vi "CheckUserFiles.vi"(8 "ErrorArray":errorcluster[](array[cluster]), 11 "Config in":refnum<class "Config.lvclass">) -> (0 "ErrorArray":errorcluster[](array[cluster]), 3 "Config out":refnum<class "Config.lvclass">)   [LabVIEW 2014, in "Framework.lvlib" / "Config.lvclass"]
uses:
  Config.lvclass
  Config.lvclass/Config.ctl
  Accessors/Read PARTF Root Directory.vi
  <userlib>/NIST/NISTErrorLib/NISTErrorLib.lvlib
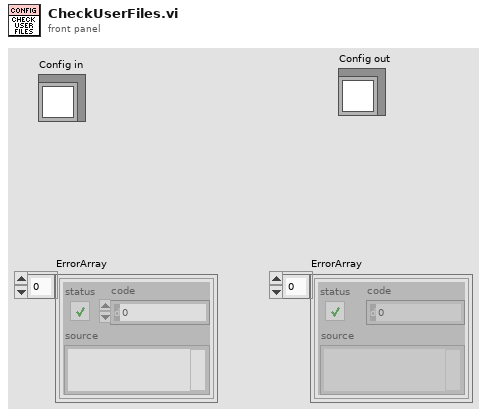
[diagram p1: front panel]
types:
  T1 = typedef "Framework.lvlib/Config.lvclass/RootDir.ctl" = cluster{"pathRootDir":path, "btnOutPath":bool, "OutDir":string, "btnOpenOutputDir":bool, "ScriptDir":string, "btnOpenScriptDir":bool, "TestDir":string, "btnOpenTestDir":bool}
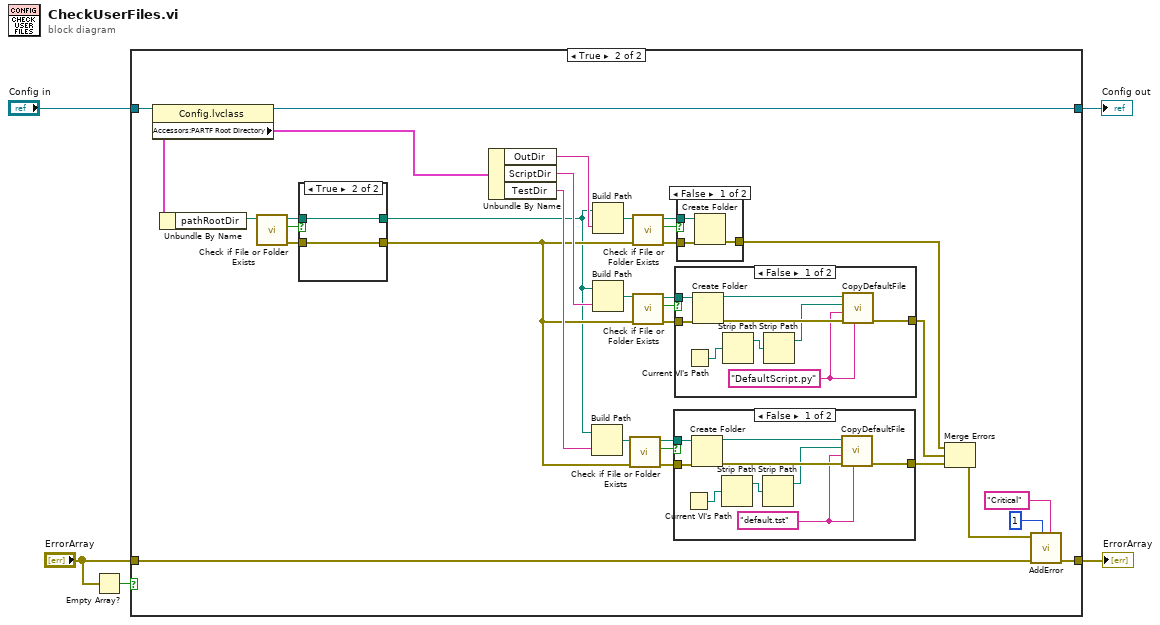
[diagram p0: block diagram]
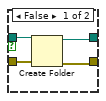
[diagram p3: hidden frame]
diagram:
  n1 = Empty Array?(array="ErrorArray") -> (empty?=w2:bool)
  n2 = case shown="True" w2 {
    tunnel: [w7 w38] -> w4
    tunnel: "Config in" -> [w7 w39]
    tunnel: "ErrorArray" -> [w6 w8]
    tunnel: [w6 w12] -> w1
    frame False {
    }
    frame True {
      n3 = property class="Config.lvclass"(reference=w39) -> (reference out=w38:refnum<class "Config.lvclass">, "Accessors:PARTF Root Directory"=w37:T1)  [unwired: 1 in, 1 out]
      n4 = Unbundle By Name(w37) -> ("pathRootDir"=w36:path)
      n5 = call <vilib>:"Check if File or Folder Exists.vi"("path"=w36) -> ("error out"=w16:errorcluster, "file or folder exists?"=w18:bool, "dup path"=w17:path)  [unwired: 8 in]
      n6 = case shown="True" w18 {
        tunnel: w17 -> [w42 w44]
        tunnel: w16 -> [w43 w45]
        tunnel: [w40 w45] -> w15
        tunnel: [w41 w44] -> w14
        frame False {
          n7 = Create Folder(path (use dialog)=w42, error in=w43) -> (created path=w41:path, error out=w40:errorcluster)  [unwired: 1 in, 1 out]
        }
        frame True {
        }
      }
      n8 = Unbundle By Name(w37) -> ("OutDir"=w35:string, "ScriptDir"=w34:string, "TestDir"=w33:string)
      n9 = Build Path(base path=w14, name or relative path=w33) -> (appended path=w30:path)
      n10 = Build Path(base path=w14, name or relative path=w35) -> (appended path=w32:path)
      n11 = Build Path(base path=w14, name or relative path=w34) -> (appended path=w31:path)
      n12 = call <vilib>:"Check if File or Folder Exists.vi"("error in (no error)"=w15, "path"=w30) -> ("error out"=w22:errorcluster, "file or folder exists?"=w13:bool, "dup path"=w23:path)  [unwired: 7 in]
      n13 = call <vilib>:"Check if File or Folder Exists.vi"("error in (no error)"=w15, "path"=w32) -> ("error out"=w27:errorcluster, "file or folder exists?"=w29:bool, "dup path"=w28:path)  [unwired: 7 in]
      n14 = call <vilib>:"Check if File or Folder Exists.vi"("error in (no error)"=w15, "path"=w31) -> ("error out"=w25:errorcluster, "file or folder exists?"=w24:bool, "dup path"=w26:path)  [unwired: 7 in]
      n15 = case shown="False" w13 {
        tunnel: w23 -> [w53 _]
        tunnel: w22 -> [w54 w55]
        tunnel: [w46 w55] -> w21
        frame False {
          w47 = "default.tst"
          n16 = Current VI's Path() -> (path=w51:path)
          n17 = Create Folder(path (use dialog)=w53, error in=w54) -> (created path=w49:path, error out=w50:errorcluster)  [unwired: 1 in, 1 out]
          n18 = Strip Path(path=w51) -> (stripped path=w52:path)  [unwired: 1 out]
          n19 = Strip Path(path=w52) -> (stripped path=w48:path)  [unwired: 1 out]
          n20 = call "CopyDefaultFile.vi"("OriginFile"=w47, "error in (no error)"=w50, "DestFile"=w47, "Origin"=w48, "Destination"=w49) -> ("error out"=w46:errorcluster)  [unwired: 6 in]
        }
        frame True {
        }
      }
      n21 = case shown="False" w24 {
        tunnel: w26 -> [w63 _]
        tunnel: w25 -> [w64 w65]
        tunnel: [w56 w65] -> w20
        frame False {
          w59 = "DefaultScript.py"
          n22 = Current VI's Path() -> (path=w61:path)
          n23 = Create Folder(path (use dialog)=w63, error in=w64) -> (created path=w58:path, error out=w60:errorcluster)  [unwired: 1 in, 1 out]
          n24 = Strip Path(path=w61) -> (stripped path=w62:path)  [unwired: 1 out]
          n25 = Strip Path(path=w62) -> (stripped path=w57:path)  [unwired: 1 out]
          n26 = call "CopyDefaultFile.vi"("OriginFile"=w59, "error in (no error)"=w60, "DestFile"=w59, "Origin"=w57, "Destination"=w58) -> ("error out"=w56:errorcluster)  [unwired: 6 in]
        }
        frame True {
        }
      }
      n27 = case shown="False" w29 {
        tunnel: w28 -> [w67 _]
        tunnel: w27 -> [w68 w69]
        tunnel: [w66 w69] -> w19
        frame False {
          n28 = Create Folder(path (use dialog)=w67, error in=w68) -> (error out=w66:errorcluster)  [unwired: 1 in, 2 out]
        }
        frame True {
        }
      }
      n29 = Merge Errors(w19, w20, w21) -> (w9:errorcluster)
      n30 = call <userlib>:"AddError.vi"("Severity"="Critical", "Priority"=u8 1, "ErrorArray"=w8, "error in (no error)"=w9) -> ("ErrorArray"=w12:errorcluster[])  [unwired: 6 in, 1 out]
    }
  }
  "Config out" <- w4
  "ErrorArray" <- w1
